vi "Query UUT Details.vi"(8 "error in":errorcluster, 10 "Name_Request":refnum<notifier>, 11 "Base Software in":refnum<class "Base Software.lvclass">) -> (0 "error out":errorcluster, 3 "Base Software out":refnum<class "Base Software.lvclass">)   [LabVIEW 2019, in "Base Software.lvlib" / "Main.lvlib" / "Base Software.lvclass"]
uses:
  Project/Base Software.lvclass
  Accessors/Indicators/Read Model.vi
  Accessors/Indicators/Read Serial.vi
  Accessors/Indicators/Read Operator.vi
  Accessors/Indicators/Read Witness.vi
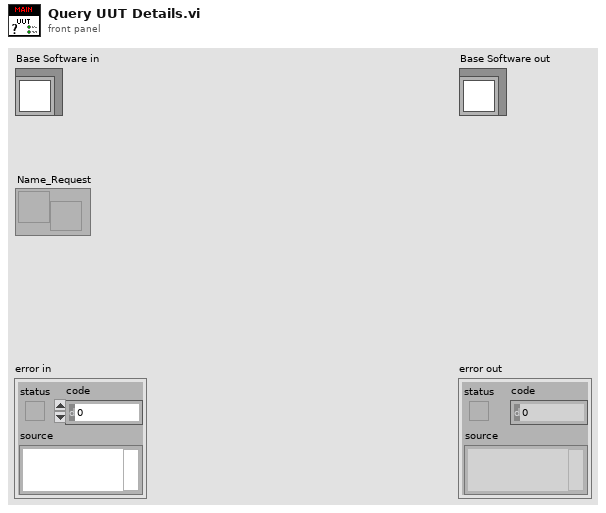
[diagram p1: front panel]
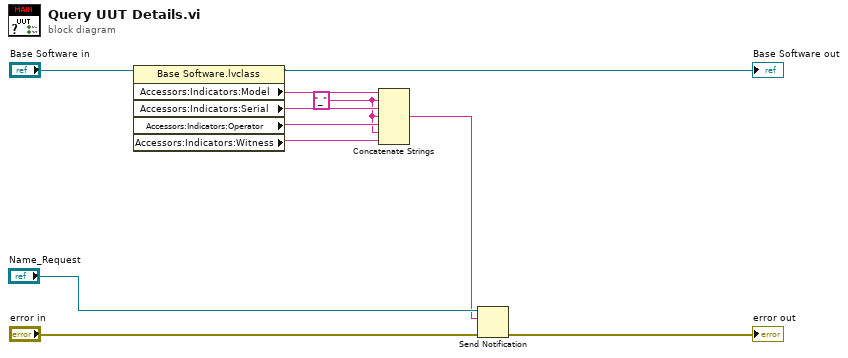
[diagram p0: block diagram]
diagram:
  w7 = "_"
  n1 = property class="Base Software.lvclass"(reference="Base Software in") -> (reference out=→"Base Software out":refnum<class "Base Software.lvclass">, "Accessors:Indicators:Model"=w10:string, "Accessors:Indicators:Serial"=w9:string, "Accessors:Indicators:Operator"=w8:string, "Accessors:Indicators:Witness"=w6:string)  [unwired: 1 in, 1 out]
  n2 = Concatenate Strings(w10, w7, w9, w7, w8, w7, w6) -> (w1:string)
  n3 = Send Notification(notification=w1, notifier="Name_Request", error in (no error)="error in") -> (error out=→"error out":errorcluster)  [unwired: 1 out]
